vi "choose status.vi"(8 "error in":errorcluster, 10 "status in":T1=enum."Setup", 11 "Controls":T2) -> (0 "error out":errorcluster, 3 "status out":T1)   [LabVIEW 2015]
uses:
  controls/state.ctl
panel:
  # "Continuous"
  # "Single"
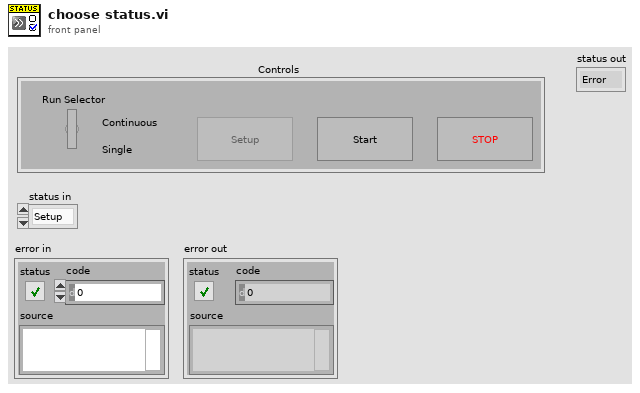
[diagram p1: front panel]
types:
  T1 = typedef "state.ctl" = enum16{"Error", "End", "Start", "Exit", "Setup", "Low pressure", "Rain", "Run", "Idle", "Initialize"}
  T2 = cluster{"Run Selector":bool, "Setup":bool, "Start":bool, "Stop":bool}
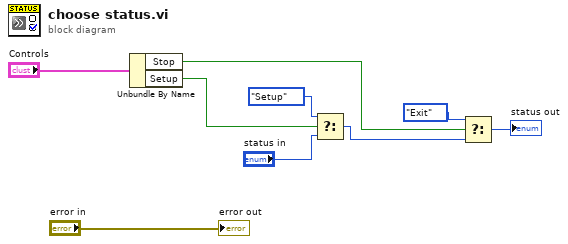
[diagram p0: block diagram]
diagram:
  n1 = Unbundle By Name("Controls") -> ("Stop"=w6:bool, "Setup"=w4:bool)
  n2 = Select(t=state."Setup" ("status"), s=w4, f="status in") -> (s? t:f=w7:T1)
  n3 = Select(t=state."Exit", s=w6, f=w7) -> (s? t:f=→"status out":T1)
  "error out" <- "error in"
